vi "DeadReckoning.vi"() -> ()   [LabVIEW 2024]
panel:
  in  "Frequency":dbl format="%#_13g"
  in  "Spd(kph)":dbl(slide) scale=0.0..15.0
  in  "Steer":dbl(slide) scale=-20.0..20.0
  in  "stop":bool
  out "XY Graph":cluster{dbl[], dbl[]}(graph)
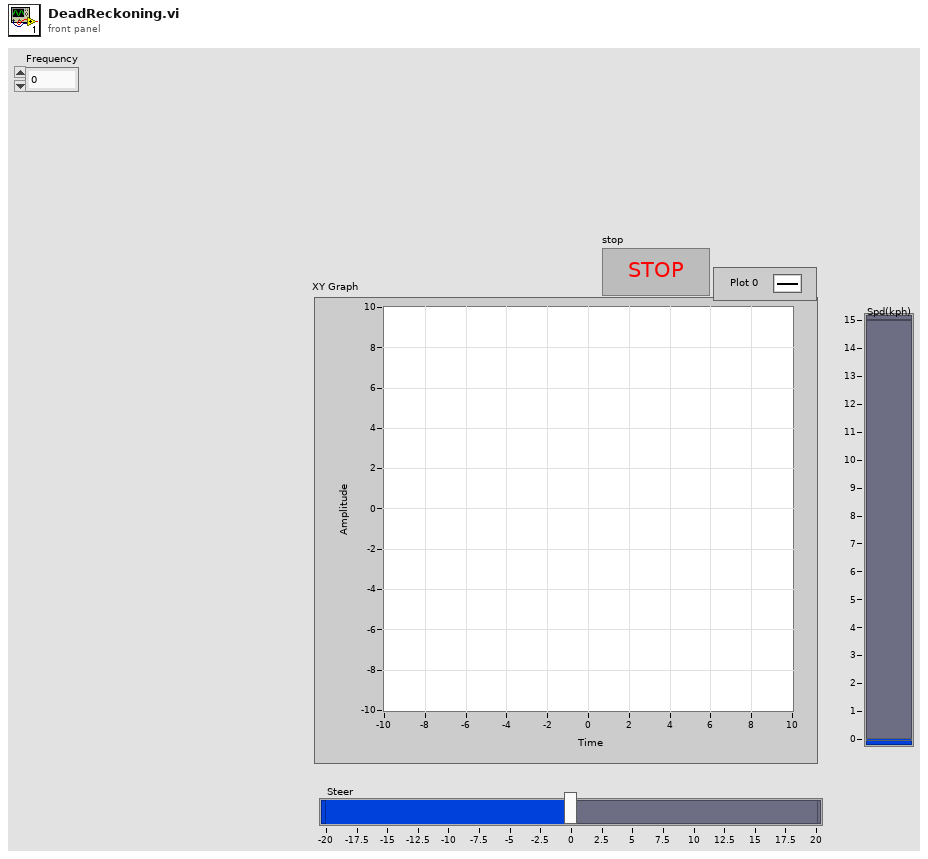
[diagram p1: front panel]
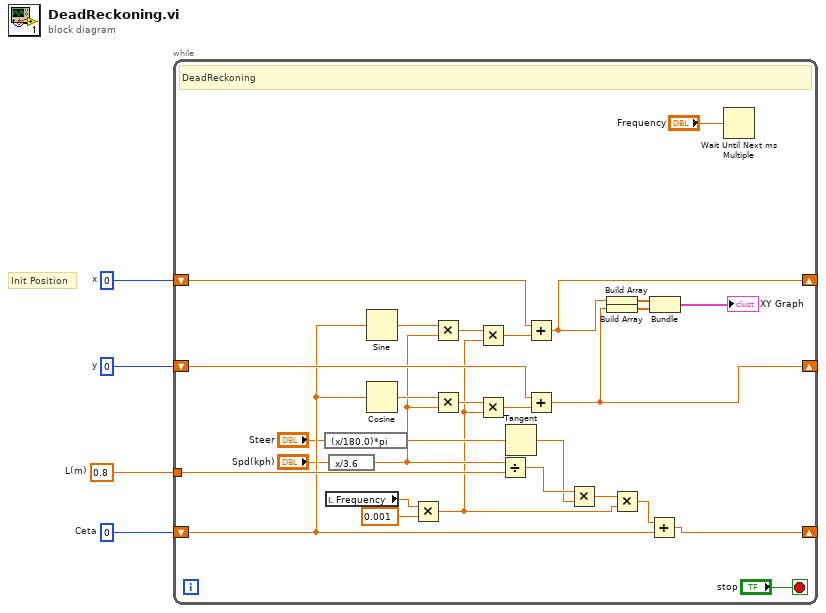
[diagram p0: block diagram]
diagram:
  w3 = 0  # Ceta
  w1 = 0  # x
  w2 = 0  # y
  w4 = 0.8  # L(m)
  # "Init Position"
  n1 = while {
    tunnel: w4 -> [w33]
    shift-right: [w15] -> _
    shift-left: w3 -> [w17]
    shift-right: [w20] -> _
    shift-left: w1 -> [w24]
    shift-right: [w19] -> _
    shift-left: w2 -> [w25]
    stop <- "stop" stop-if-true
    # "DeadReckoning"
    n2 = expression code="(x/180.0)*pi" ("degrees to radians")("Steer") -> (w12:dbl)
    n3 = local read "Frequency"() -> (w5:dbl)
    n4 = expression code="x/3.6" ("k/h to m/s")("Spd(kph)") -> (w10:dbl)
    n5 = Sine(x=w17) -> (sin(x)=w30:dbl)
    n6 = Cosine(x=w17) -> (cos(x)=w31:dbl)
    n7 = Multiply(x=w5, y=0.001) -> (x*y=w6:dbl)
    n8 = Multiply(x=w30, y=w10) -> (x*y=w29:dbl)
    n9 = Multiply(x=w31, y=w10) -> (x*y=w28:dbl)
    n10 = Multiply(x=w29, y=w6) -> (x*y=w27:dbl)
    n11 = Multiply(x=w28, y=w6) -> (x*y=w26:dbl)
    n12 = Divide(x=w10, y=w33) -> (x/y=w32:dbl)
    n13 = Tangent(1:w12) -> (0:w13:dbl)
    n14 = Add(x=w24, y=w27) -> (x+y=w20:dbl)
    n15 = Add(x=w25, y=w26) -> (x+y=w19:dbl)
    n16 = Multiply(x=w32, y=w13) -> (x*y=w14:dbl)
    n17 = Build Array(w20) -> (w23:dbl[])
    n18 = Build Array(w19) -> (w22:dbl[])
    n19 = Multiply(x=w14, y=w6) -> (x*y=w16:dbl)
    n20 = Add(x=w16, y=w17) -> (x+y=w15:dbl)
    n21 = Bundle(w23, w22) -> (→"XY Graph":cluster{dbl[], dbl[]})  [unwired: 1 in]
    n22 = Wait Until Next ms Multiple(millisecond multiple="Frequency") -> ()  [unwired: 1 out]
  }
